vi "Set Unit ID.vi"(8 "error in":errorcluster, 10 "unit ID":u8, 11 "Modbus master in":refnum<class "Modbus Master.lvclass">) -> (0 "error out":errorcluster, 3 "Modbus master out":refnum<class "Modbus Master.lvclass">)   [LabVIEW 2015, in "Modbus Library.lvlib" / "Modbus Master.lvclass"]
doc: "Provides a simple function for defining the <B>unit ID</B> which is the target of Modbus master read and write operations. This function takes effect immediately, and will change the target of any future operations using the instance returned by <B>Modbus master out</B>. Multiple units can be accessed simultaneously by forking the wire. This function only applies when using the RTU or ASCII serial transmission data unit. The TCP/IP transmission data unit ignores the unit ID."
uses:
  Modbus Master.lvclass
  Modbus API.lvclass/Modbus API.ctl
  Transmission Data Unit/Transmission Data Unit.lvclass/Transmission Data Unit.ctl
  Transmission Data Unit/Transmission Data Unit.lvclass
  Modbus API.lvclass
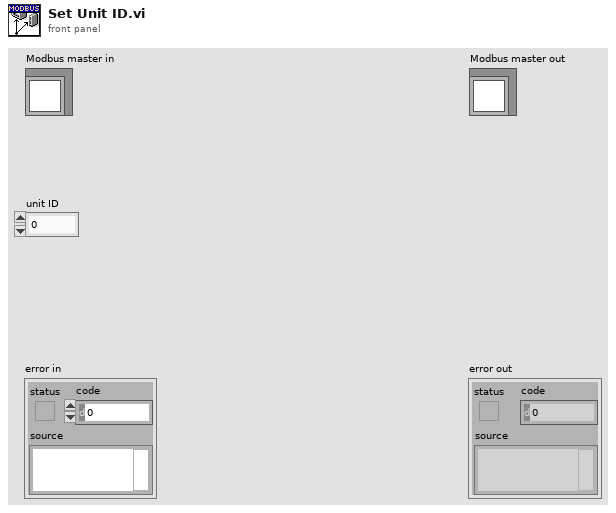
[diagram p1: front panel]
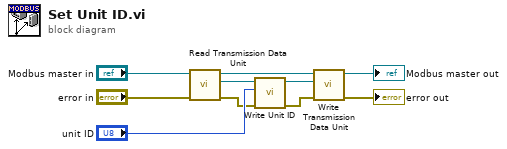
[diagram p0: block diagram]
diagram:
  n1 = call "Read Transmission Data Unit.vi"("error in"="error in", "Modbus instance in"="Modbus master in") -> ("error out"=w3:errorcluster, "transmission data unit"=w6:refnum<class "Transmission Data Unit.lvclass">, "Modbus instance out"=w8:refnum<class "Modbus Master.lvclass">)  [unwired: 7 in]
  n2 = call "Write Unit ID.vi"("error in"=w3, "unit ID"="unit ID", "transmission data unit in"=w6) -> ("error out"=w4:errorcluster, "transmission data unit out"=w5:refnum<class "Transmission Data Unit.lvclass">)  [unwired: 7 in]
  n3 = call "Write Transmission Data Unit.vi"("error in"=w4, "transmission data unit"=w5, "Modbus instance in"=w8) -> ("error out"=→"error out":errorcluster, "Modbus instance out"=→"Modbus master out":refnum<class "Modbus Master.lvclass">)  [unwired: 7 in]
